vi "setDetails.vi"(8 "error in (no error)":errorcluster, 10 "details":T2, 11 "reference in":refnum<class "peapod.lvclass">) -> (0 "error out":errorcluster, 3 "reference out":refnum<class "peapod.lvclass">)   [LabVIEW 2014, in "peapod.lvclass"]
uses:
  peapod.lvclass
  SYS/Devices Controller_llb/deviceType.ctl
  SYS/Devices Controller_llb/Devices Controller.lvclass
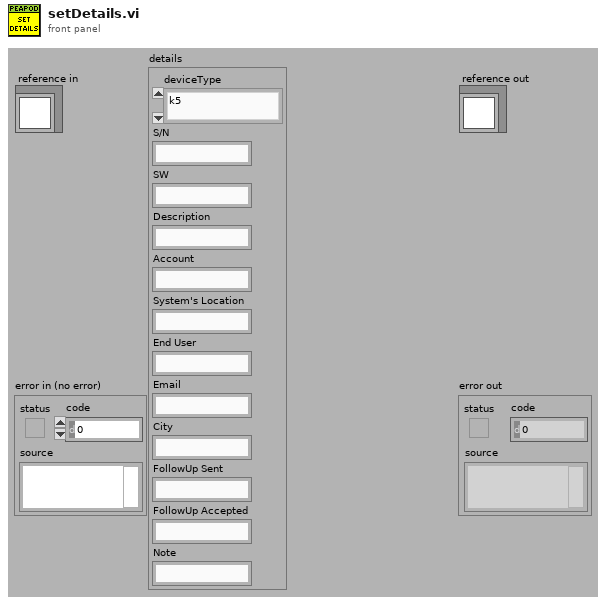
[diagram p1: front panel]
types:
  T1 = typedef "Devices Controller.lvclass/deviceType.ctl" = enum16{"k5", "k4b2", "fitmate", "cpet", "rmr", "bodyBoxPft", "bp", "pp"}
  T2 = cluster{"deviceType":T1, "S/N":string, "SW":string, "Description":string, "Account":string, "System's Location":string, "End User":string, "Email":string, "City":string, "FollowUp Sent":string, "FollowUp Accepted":string, "Note":string}
  T3 = typedef "peapod.lvclass/ObjectAttributesRef.ctl" = refnum<data-value>
  T4 = typedef "peapod.lvclass/ObjectAttributes.ctl" = cluster{"MyAttribute":dbl, "details":cluster{"deviceType":T1, "S/N":string, "SW":string, "Description":string, "Account":string, "System's Location":string, "End User":string, "Email":string, "City":string, "FollowUp Sent":string, "FollowUp Accepted":string, "Note":string}}
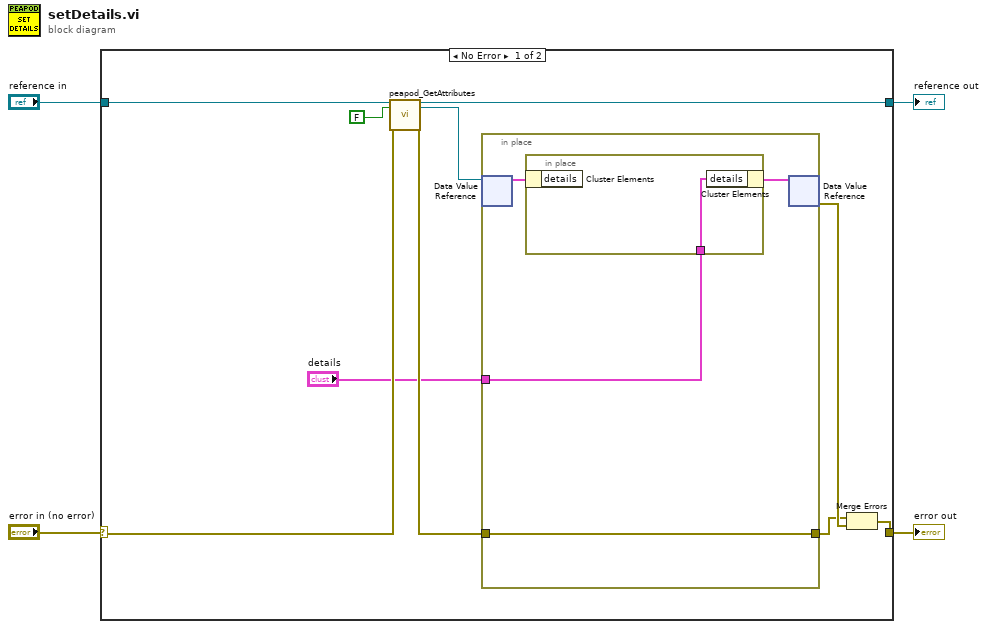
[diagram p0: block diagram]
diagram:
  n1 = case shown="No Error" "error in (no error)" {
    selector: "error in (no error)" -> [w9 w21]
    tunnel: [w14 w21] -> w3
    tunnel: [w7 w20] -> w1
    tunnel: "reference in" -> [w11 w20]
    frame No Error {
      n2 = call "peapod_GetAttributes.vi"("reference in"=w11, "return data? (T)"=FALSE, "error in (no error)"=w9) -> ("reference out"=w7:refnum<class "peapod.lvclass">, "attributes ref"=w6:T3, "error out"=w8:errorcluster)  [unwired: 13 in, 1 out]
      n3 = in-place {
        in-place-border: w8 -> [w16]
        in-place-border: [w16] -> w12
        in-place-border: "details" -> [w15]
        n4 = in-place-dvr #1(w6) -> (w17:T4)  [unwired: 1 out]
        n5 = in-place {
          in-place-border: w15 -> [w19]
          n6 = in-place-cluster #2(w17) -> ()  [unwired: 1 out]
          n7 = in-place-cluster #2("details"=w19) -> (w18:T4)
        }
        n8 = in-place-dvr #1(w18) -> (w13:errorcluster)  [unwired: 1 out]
      }
      n9 = Merge Errors(w12, w13) -> (w14:errorcluster)
    }
    frame Error {
    }
  }
  "error out" <- w3
  "reference out" <- w1
